vi "registerStopEvent.vi"(8 "error in (no error)":errorcluster, 11 "MonoPubSubData in":refnum<class "MonoPubSubData.lvclass">) -> (0 "error out":errorcluster, 2 "stopRegs":refnum<event-registration>, 3 "MonoPubSubData out":refnum<class "MonoPubSubData.lvclass">)   [LabVIEW 2016, in "MonoPubSubData.lvclass"]
uses:
  MonoPubSubData.lvclass
  MonoPubSubData.lvclass/MonoPubSubData.ctl
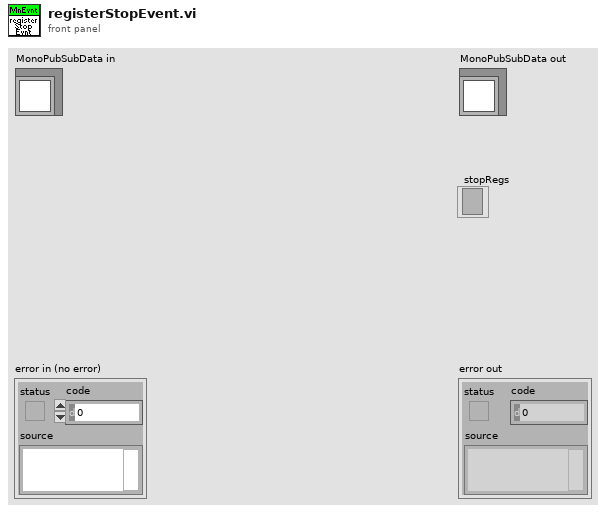
[diagram p1: front panel]
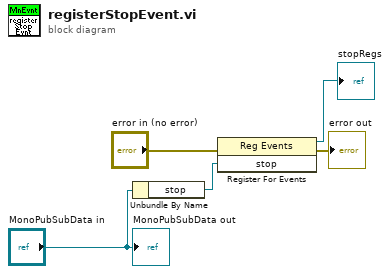
[diagram p0: block diagram]
diagram:
  n1 = Unbundle By Name("MonoPubSubData in") -> ("stop"=w2:refnum<user-event>)
  n2 = register-events(error in="error in (no error)", w2) -> (reference out=→"stopRegs":refnum<event-registration>, error out=→"error out":errorcluster)  [unwired: 1 in]
  "MonoPubSubData out" <- "MonoPubSubData in"
